vi "Finish Defrag.vi"(8 "Cancelled":bool, 9 "Temp":path, 10 "Original":path) -> ()   [LabVIEW 2019, in "TDMS.lvlib" / "TDMS.lvclass"]
uses:
  TDMS.lvclass
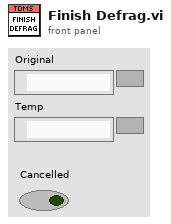
[diagram p1: front panel]
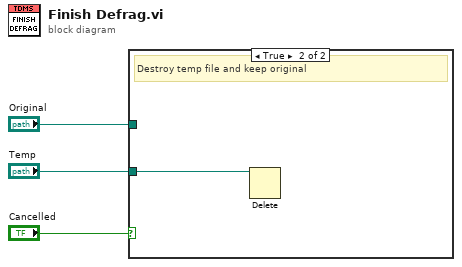
[diagram p0: block diagram]
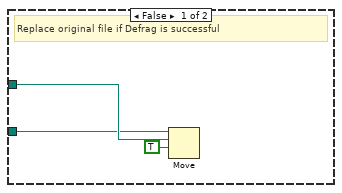
[diagram p2: hidden frame]
diagram:
  n1 = case shown="True" "Cancelled" {
    tunnel: "Original" -> [w6 _]
    tunnel: "Temp" -> [w5 w7]
    frame False {
      # "Replace original file if Defrag is successful"
      n2 = Move(source path=w5, 9:TRUE ("overwrite (F)"), 10:w6) -> ()  [unwired: 2 in, 3 out]
    }
    frame True {
      # "Destroy temp file and keep original"
      n3 = Delete(path (use dialog)=w7) -> ()  [unwired: 4 in, 3 out]
    }
  }
